vi "COP Message Interpreter.vi"() -> ()   [LabVIEW 2009]
uses:
  Support Files/JUDP Read Queue Element.ctl
  Support Files/Address.ctl
  Support Files/JUDP Write Queue Element.ctl
  Support Files/ServiceRec.ctl
  cRIO/Functional Global Variables/Actions for FG's.ctl
  Support Files/JAUS Controller.ctl
panel:
  out "Message Code":u16 format="%.0x"
  out "HB":bool
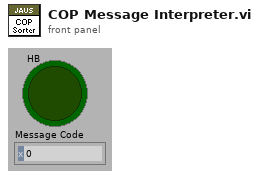
[diagram p1: front panel]
types:
  T1 = typedef "ServiceRec.ctl" = cluster{"ServiceURI":string, "MajorVerNum":u8, "MinorVerNum":u8}
  T2 = typedef "JUDP Write Queue Element.ctl" = cluster{"Encoded JAUS Message":string, "Destination ID":u32}
  T3 = typedef "JUDP Read Queue Element.ctl" = cluster{"Payload":string, "Sender ID":T4, "Command Code":u16}
  T4 = typedef "Address.ctl" = cluster{"Subsystem Id":u16, "Node Id":u8, "Component Id":u8}
  T5 = typedef "Actions for FG's.ctl" = enum16{"Read", "Write"}
  T6 = typedef "JAUS Controller.ctl" = cluster{"ID":T4, "Authority Code":u8}
  T7 = typedef "LocalPose.ctl" = cluster{" X":dbl, " Y":dbl, " Z":dbl, "Position RMS":dbl, "Roll":dbl, "Pitch":dbl, "Yaw":dbl, "Attitude RMS":dbl, "TimeRec":T8}
  T8 = typedef "TimeRec.ctl" = cluster{"Milliseconds":u32, "Seconds":u32, "Minutes":u32, "Hours":u32, "Day":u32}
  T9 = typedef "VelocityState.ctl" = cluster{"Velocity X":dbl, "Velocity Y":dbl, "Velocity Z":dbl, "Velocity RMS":dbl, "Roll Rate":dbl, "Pitch Rate":dbl, "Yaw Rate":dbl, "Rate RMS":dbl, "TimeRec":T8}
  T10 = typedef "RequestIDRec.ctl" = cluster{"RequestId":u8, "Element List":T11[]}
  T11 = typedef "ElementRec.ctl" = cluster{"ElementUID":u16, " PreviousUID":u16, " NextUID":u16, "LocalWaypointRec":T12}
  T12 = typedef "LocalWaypointRec.ctl" = cluster{"Presence Vector":u8, " X":dbl, " Y":dbl, " Z":dbl, "Roll":dbl, "Pitch":dbl, "Yaw":dbl, "Waypoint Tolerance":dbl, "Path Tolerance":dbl, "Is Active?":bool}
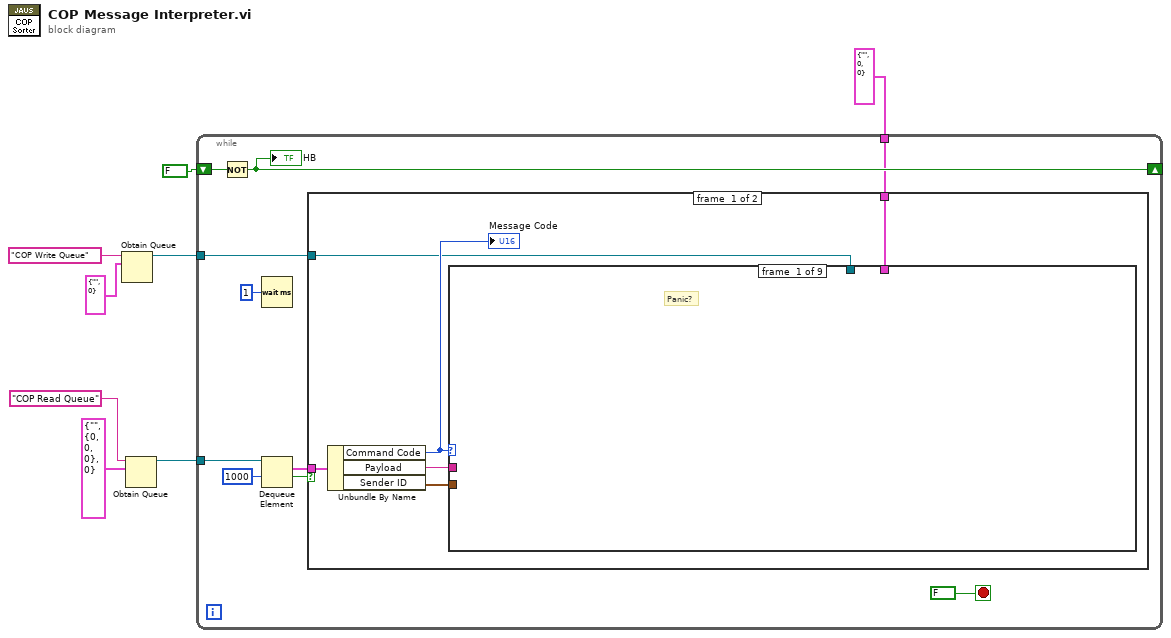
[diagram p0: block diagram]
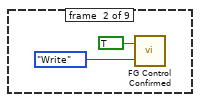
[diagram p2: hidden frame]
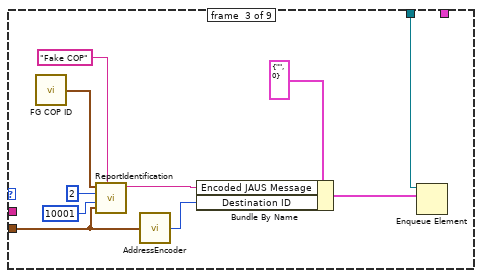
[diagram p3: hidden frame]
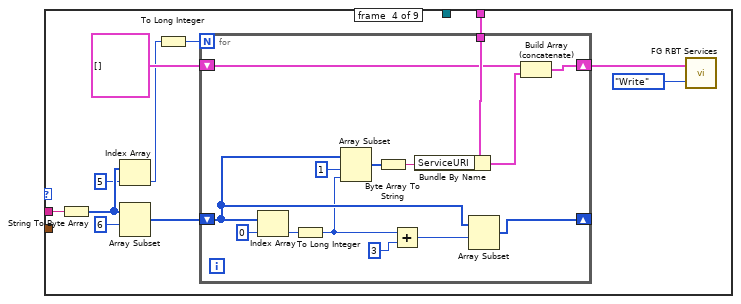
[diagram p4: hidden frame]
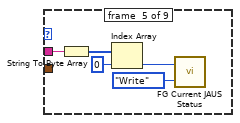
[diagram p5: hidden frame]
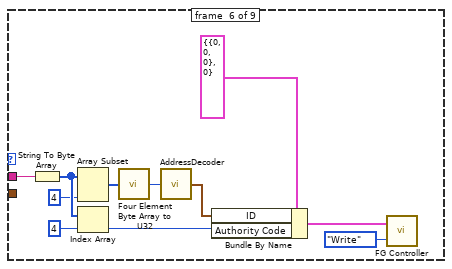
[diagram p6: hidden frame]
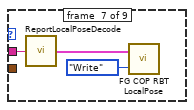
[diagram p7: hidden frame]
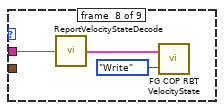
[diagram p8: hidden frame]
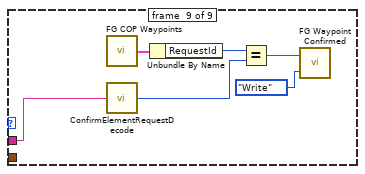
[diagram p9: hidden frame]
diagram:
  n1 = Obtain Queue(name (unnamed)="COP Write Queue", element data type=T2 {"Encoded JAUS Message"="", "Destination ID"=0} ("Cluster")) -> (queue out=w2:refnum<queue>)  [unwired: 3 in, 2 out]
  n2 = Obtain Queue(name (unnamed)="COP Read Queue", element data type=T3 {"Payload"="", "Sender ID"={"Subsystem Id"=0, "Node Id"=0, "Component Id"=0}, "Command Code"=0} ("Receive FSM Queue Element")) -> (queue out=w6:refnum<queue>)  [unwired: 3 in, 2 out]
  n3 = while {
    tunnel: w6 -> [w18]
    shift-right: [w12] -> _
    shift-left: FALSE ("timed out?") -> [w13]
    tunnel: w2 -> [w10]
    tunnel: T1 {"ServiceURI"="", "MajorVerNum"=0, "MinorVerNum"=0} ("ServiceRec") -> [w9]
    stop <- FALSE stop-if-true
    n4 = Not(x=w13) -> (.not. x?=w12:bool)
    "HB" <- w12
    n5 = Wait (ms)(milliseconds to wait=u32 1) -> ()  [unwired: 1 out]
    n6 = Dequeue Element(queue=w18, timeout in ms (-1)=1000) -> (element=w16:T3, timed out?=w15:bool)  [unwired: 1 in, 2 out]
    n7 = case shown="False" w15 {
      tunnel: w16 -> [w24 _]
      tunnel: w10 -> [w20 _]
      tunnel: w9 -> [w19 _]
      frame #0 {
        n8 = Unbundle By Name(w24) -> ("Command Code"=w21:u16, "Payload"=w23:string, "Sender ID"=w22:T4)
        "Message Code" <- w21
        n9 = case shown="4403" w21 {
          tunnel: w23 -> [_ _ _ w45 w66 w77 w80 w83 w89]
          tunnel: w22 -> [_ _ w30 _ _ _ _ _ _]
          tunnel: w20 -> [_ _ w28 _ _ _ _ _ _]
          tunnel: w19 -> [_ _ _ w44 _ _ _ _ _]
          frame #0 {
            # "Panic?"
          }
          frame #1 {
            n10 = call "FG Control Confirmed.vi"("FG Action (Read)"=Actions_for_FG's."Write", "Control Confirmed in"=TRUE) -> ()  [unwired: 1 out]
          }
          frame #2 {
            n11 = call "FG COP ID.vi"() -> ("COP ID out"=w34:T4)  [unwired: 2 in]
            n12 = call "ReportIdentification.vi"("Vehicle Name"="Fake COP", "Destination"=w30, "Type"=u16 10001, "QueryType"=u8 2, "Source"=w34) -> ("Encoded JAUS Message"=w33:string)  [unwired: 6 in]
            n13 = call "AddressEncoder.vi"("Address Cluster"=w30) -> ("Address"=w29:u32)
            n14 = Bundle By Name(cluster=T2 {"Encoded JAUS Message"="", "Destination ID"=0} ("Cluster"), "Encoded JAUS Message"=w33, "Destination ID"=w29) -> (w32:T2)
            n15 = Enqueue Element(queue=w28, element=w32) -> ()  [unwired: 2 in, 3 out]
          }
          frame #3 {
            n16 = String To Byte Array(string=w45) -> (unsigned byte array=w42:u8[])
            n17 = Index Array(array=w42, index=5) -> (element=w40:u8)
            n18 = Array Subset(array=w42, index=6 ("length")) -> (w43:u8[])  [unwired: 1 in]
            n19 = To Long Integer(number=w40) -> (32bit integer=w39:i32)
            n20 = for {
              N: w39 -> [_]
              shift-right: [w49] -> w38
              shift-left: T1[] [] -> [w48]
              shift-right: [w60] -> _
              shift-left: w43 -> [w59]
              tunnel: w44 -> [w52]
              n21 = Index Array(array=w59, index=0) -> (element=w58:u8)
              n22 = To Long Integer(number=w58) -> (32bit integer=w56:i32)
              n23 = Array Subset(array=w59, index=1, length=w56) -> (w55:u8[])
              n24 = Byte Array To String(unsigned byte array=w55) -> (string=w51:string)
              n25 = Add(x=w56, y=3) -> (x+y=w54:i32)
              n26 = Bundle By Name(cluster=w52, "ServiceURI"=w51) -> (w50:T1)
              n27 = Array Subset(array=w59, index=w54) -> (w60:u8[])  [unwired: 1 in]
              n28 = Build Array (concatenate)(w48, w50) -> (w49:T1[])
            }
            n29 = call "FG RBT Services.vi"("FG Action (Read)"=Actions_for_FG's."Write", "Services in"=w38) -> ()  [unwired: 1 out]
          }
          frame #4 {
            n30 = String To Byte Array(string=w66) -> (unsigned byte array=w65:u8[])
            n31 = Index Array(array=w65, index=0) -> (element=w63:u8)
            n32 = call "FG Current JAUS Status.vi"("FG Action (Read)"=Actions_for_FG's."Write", "Status in"=w63) -> ()  [unwired: 1 out]
          }
          frame #5 {
            n33 = String To Byte Array(string=w77) -> (unsigned byte array=w70:u8[])
            n34 = Array Subset(array=w70, length=4) -> (w68:u8[])  [unwired: 1 in]
            n35 = Index Array(array=w70, index=4) -> (element=w72:u8)
            n36 = call "Four Element Byte Array to U32.vi"("Four Element Byte Array"=w68) -> ("U32 out"=w67:u32)
            n37 = call "AddressDecoder.vi"("Address"=w67) -> ("Address Cluster"=w75:T4)
            n38 = Bundle By Name(cluster=T6 {"ID"={"Subsystem Id"=0, "Node Id"=0, "Component Id"=0}, "Authority Code"=0} ("Controller in"), "ID"=w75, "Authority Code"=w72) -> (w74:T6)
            n39 = call "FG Controller.vi"("FG Action (Read)"=Actions_for_FG's."Write", "Controller in"=w74) -> ()  [unwired: 1 out]
          }
          frame #6 {
            n40 = call "ReportLocalPoseDecode.vi"("Payload"=w80) -> ("LocalPose"=w78:T7)
            n41 = call "FG COP RBT LocalPose.vi"("FG Action (Read)"=Actions_for_FG's."Write", "RBT LocalPose in"=w78) -> ()  [unwired: 1 out]
          }
          frame #7 {
            n42 = call "ReportVelocityStateDecode.vi"("Payload"=w83) -> ("VelocityState"=w82:T9)
            n43 = call "FG COP RBT VelocityState.vi"("FG Action (Read)"=Actions_for_FG's."Write", "RBT VelocityState in"=w82) -> ()  [unwired: 1 out]
          }
          frame #8 {
            n44 = call "FG COP Waypoints.vi"() -> ("COP Waypoints out"=w88:T10)  [unwired: 2 in]
            n45 = call "ConfirmElementRequestDecode.vi"("Payload"=w89) -> ("RequestId"=w86:u8)
            n46 = Unbundle By Name(w88) -> ("RequestId"=w87:u8)
            n47 = Equal?(x=w87, y=w86) -> (x = y?=w85:bool)
            n48 = call "FG Waypoint Confirmed.vi"("FG Action (Read)"=Actions_for_FG's."Write", "Waypoints \nConfirmed In"=w85) -> ()  [unwired: 1 out]
          }
        }
      }
      frame #1 {
      }
    }
  }
